vi "Axsun OCT Control Example.vi"() -> ()   [LabVIEW 2018]
uses:
  C:/Projects/Serial Sectioning OCT - TortoiseGIT/SerialSectOCT/Software/Hardware Mfg/Axsun Laser/AxsunOCTControl.dll
  AxsunOCTControl.dll
panel:
  in  "Reg Value (write)":u32 format="%04x"
  out "Reg Value (read)":u16 format="%04x"
  in  "Reg Number":u32
  in  "Write FPGA Register":bool
  in  "Read FPGA Register":bool
  out "Devices":string[](array[string])
  in  "Laser Off":bool
  in  "Laser On":bool
  in  "stop":bool
  out "Error":errorcluster
  out "Version":string
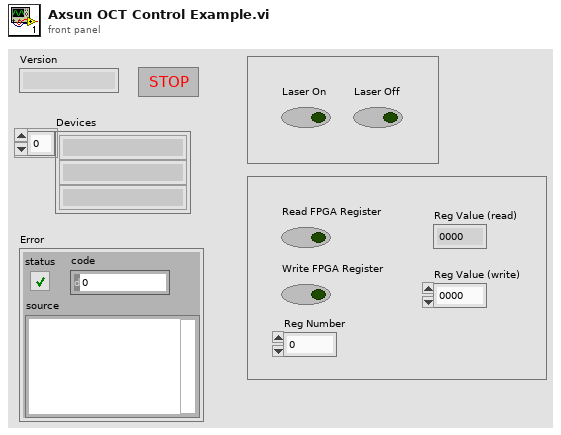
[diagram p1: front panel]
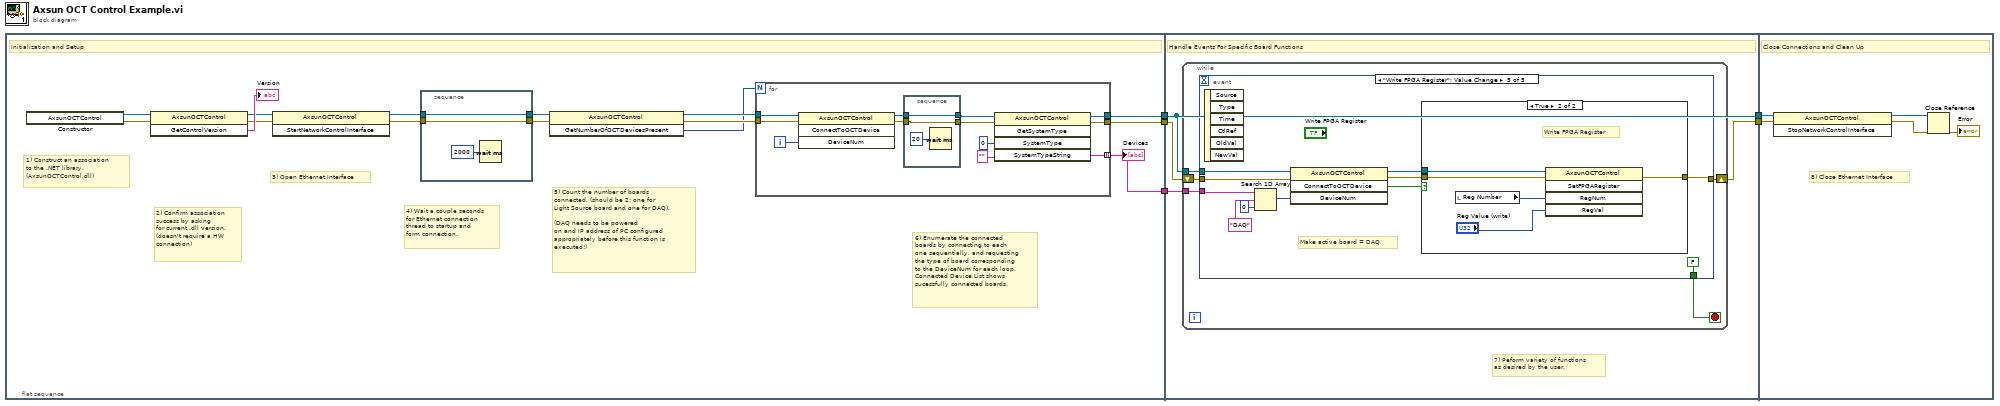
[diagram p0: block diagram]
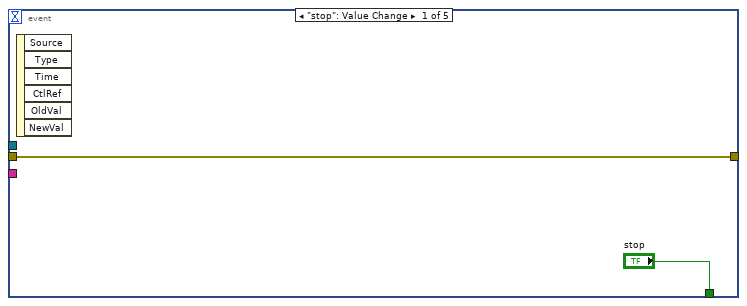
[diagram p2: hidden frame]
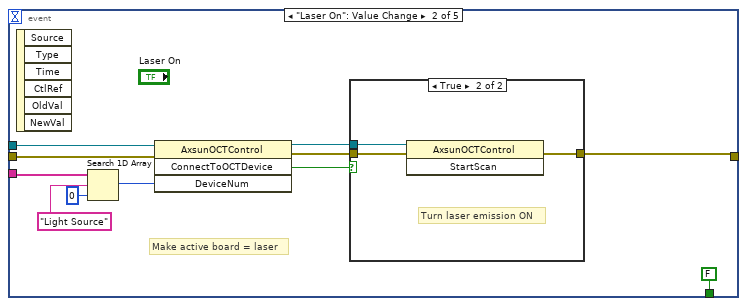
[diagram p3: hidden frame]
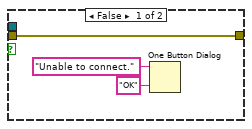
[diagram p4: hidden frame]
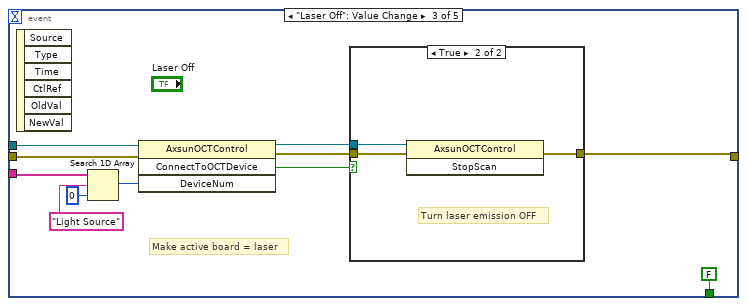
[diagram p5: hidden frame]
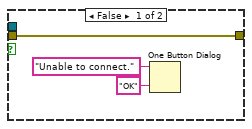
[diagram p6: hidden frame]
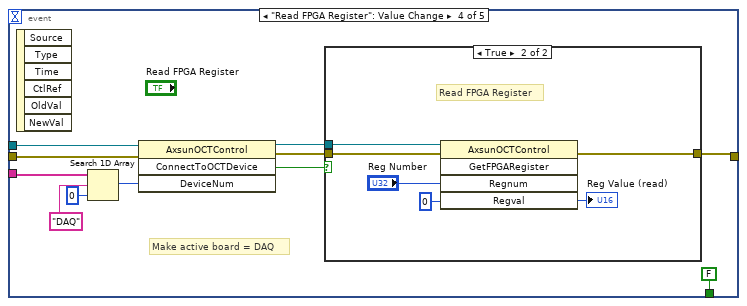
[diagram p7: hidden frame]
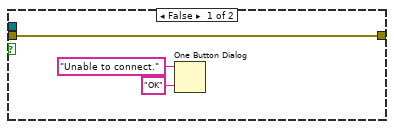
[diagram p8: hidden frame]
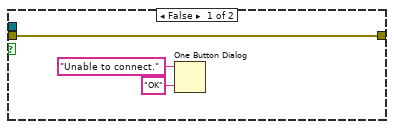
[diagram p9: hidden frame]
diagram:
  n1 = flat-sequence {
    tunnel: [w11] -> w5
    tunnel: [w10] -> w4
    tunnel: [w9] -> w2
    tunnel: w5 -> [w42]
    tunnel: w4 -> [w41]
    tunnel: [w41] -> w3
    tunnel: w2 -> [w40]
    tunnel: [w39] -> w1
    tunnel: w3 -> [w127]
    tunnel: w1 -> [w123]
    frame #0 {
      # "6) Enumerate the connected\nboards by connecting to each\none sequentially, and requesting\nthe type of board corresponding\nto the DeviceNum for each loop.\nConnected Device List shows\nsucessfully connected boards."
      # "5) Count the number of boards\nconnected. (should be 2: one for\nLight Source board and one for DAQ).\n\n(DAQ needs to be powered\non and IP address of PC configured \nappropriately before this function is\nexecuted!)"
      # "4) Wait a couple seconds\nfor Ethernet connection\nthread to startup and\nform connection."
      # "3) Open Ethernet Interface"
      # "2) Confirm association\nsuccess by asking\nfor current .dll version.\n(doesn't require a HW\nconnection)"
      # "1) Construct an association \nto the .NET library.\n(AxsunOCTControl.dll)"
      # "Initialization and Setup"
      n2 = constructor class="AxsunOCTControl"() -> (reference out=w7:refnum<k24>, error out=w6:errorcluster)  [unwired: 3 in, 1 out]
      n3 = invoke class="AxsunOCTControl" method="GetControlVersion"(reference=w7, error in=w6) -> (reference out=w19:refnum<k24>, error out=w18:errorcluster, "GetControlVersion"=→"Version":string)  [unwired: 1 in]
      n4 = invoke class="AxsunOCTControl" method="StartNetworkControlInterface"(reference=w19, error in=w18) -> (reference out=w8:refnum<k24>, error out=w17:errorcluster)  [unwired: 1 in, 1 out]
      n5 = stacked-sequence {
        tunnel: [w38] -> w16
        tunnel: w8 -> [w38]
        tunnel: [w37] -> w15
        tunnel: w17 -> [w37]
        frame #0 {
          n6 = Wait (ms)(milliseconds to wait=u32 2000) -> ()  [unwired: 1 out]
        }
      }
      n7 = invoke class="AxsunOCTControl" method="GetNumberOfOCTDevicesPresent"(reference=w16, error in=w15) -> (reference out=w14:refnum<k24>, error out=w13:errorcluster, "GetNumberOfOCTDevicesPresent"=w12:i32)  [unwired: 1 in]
      n8 = for {
        N: w12 -> [_]
        tunnel: w14 -> [w32]
        tunnel: w13 -> [w31]
        tunnel: [w27] -> w10
        tunnel: [w26] -> w11
        tunnel: [w23] -> w9 mode=indexing
        i -> [w30]
        n9 = invoke class="AxsunOCTControl" method="ConnectToOCTDevice"(reference=w32, error in=w31, "DeviceNum"=w30) -> (reference out=w25:refnum<k24>, error out=w24:errorcluster)  [unwired: 1 in, 2 out]
        n10 = stacked-sequence {
          tunnel: w25 -> [w35]
          tunnel: [w35] -> w22
          tunnel: w24 -> [w34]
          tunnel: [w34] -> w21
          frame #0 {
            n11 = Wait (ms)(milliseconds to wait=u32 20) -> ()  [unwired: 1 out]
          }
        }
        n12 = invoke class="AxsunOCTControl" method="GetSystemType"(reference=w22, error in=w21, "SystemType"=u32 0, "SystemTypeString"="") -> (reference out=w27:refnum<k24>, error out=w26:errorcluster, "SystemTypeString"=w23:string)  [unwired: 1 in, 2 out]
      }
      "Devices" <- w9
    }
    frame #1 {
      # "7) Peform variety of functions\nas desired by the user."
      # "Handle Events For Specific Board Functions"
      n13 = while {
        tunnel: w41 -> [w47]
        tunnel: w40 -> [w44]
        shift-right: [w43] -> w39
        shift-left: w42 -> [w46]
        stop <- w45 stop-if-true
        n14 = event shown="[4] \"Write FPGA Register\": Value Change" {
          selector: _ -> [_ _ _ _ _]
          dyn-events: _ -> [_ _ _ _ _]
          timeout: _ -> [_ _ _ _ _]
          tunnel: w47 -> [_ w57 w74 w91 w111]
          tunnel: w46 -> [w48 w56 w73 w90 w110]
          tunnel: ["stop" FALSE ("stop") FALSE ("stop") FALSE ("stop") FALSE ("stop")] -> w45
          tunnel: w44 -> [_ w59 w76 w93 w113]
          tunnel: [w48 w52 w69 w86 w106] -> w43
          event "stop": Value Change {
            n15 = event-data() -> ()  [unwired: 1 in, 6 out]
          }
          event "Laser On": Value Change {
            # "Make active board = laser"
            n16 = event-data() -> ()  [unwired: 1 in, 6 out]
            n17 = Search 1D Array(1D array=w59, element="Light Source", start index (0)=0) -> (index of element=w55:i32)
            n18 = invoke class="AxsunOCTControl" method="ConnectToOCTDevice"(reference=w57, error in=w56, "DeviceNum"=w55) -> (reference out=w54:refnum<k24>, error out=w53:errorcluster, "ConnectToOCTDevice"=w51:bool)  [unwired: 1 in, 1 out]
            n19 = case shown="True" w51 {
              tunnel: w54 -> [_ w66]
              tunnel: w53 -> [w63 w65]
              tunnel: [w63 w64] -> w52
              frame False {
                n20 = One Button Dialog(message="Unable to connect.", button name ("OK")="OK") -> ()  [unwired: 1 out]
              }
              frame True {
                # "Turn laser emission ON"
                n21 = invoke class="AxsunOCTControl" method="StartScan"(reference=w66, error in=w65) -> (error out=w64:errorcluster)  [unwired: 1 in, 2 out]
              }
            }
          }
          event "Laser Off": Value Change {
            # "Make active board = laser"
            n22 = event-data() -> ()  [unwired: 1 in, 6 out]
            n23 = Search 1D Array(1D array=w76, element="Light Source", start index (0)=0) -> (index of element=w72:i32)
            n24 = invoke class="AxsunOCTControl" method="ConnectToOCTDevice"(reference=w74, error in=w73, "DeviceNum"=w72) -> (reference out=w71:refnum<k24>, error out=w70:errorcluster, "ConnectToOCTDevice"=w68:bool)  [unwired: 1 in, 1 out]
            n25 = case shown="True" w68 {
              tunnel: w71 -> [_ w83]
              tunnel: w70 -> [w80 w82]
              tunnel: [w80 w81] -> w69
              frame False {
                n26 = One Button Dialog(message="Unable to connect.", button name ("OK")="OK") -> ()  [unwired: 1 out]
              }
              frame True {
                # "Turn laser emission OFF"
                n27 = invoke class="AxsunOCTControl" method="StopScan"(reference=w83, error in=w82) -> (error out=w81:errorcluster)  [unwired: 1 in, 2 out]
              }
            }
          }
          event "Read FPGA Register": Value Change {
            # "Make active board = DAQ"
            n28 = event-data() -> ()  [unwired: 1 in, 6 out]
            n29 = Search 1D Array(1D array=w93, element="DAQ", start index (0)=0) -> (index of element=w89:i32)
            n30 = invoke class="AxsunOCTControl" method="ConnectToOCTDevice"(reference=w91, error in=w90, "DeviceNum"=w89) -> (reference out=w88:refnum<k24>, error out=w87:errorcluster, "ConnectToOCTDevice"=w85:bool)  [unwired: 1 in, 1 out]
            n31 = case shown="True" w85 {
              tunnel: w88 -> [_ w103]
              tunnel: w87 -> [w97 w102]
              tunnel: [w97 w101] -> w86
              frame False {
                n32 = One Button Dialog(message="Unable to connect.", button name ("OK")="OK") -> ()  [unwired: 1 out]
              }
              frame True {
                # "Read FPGA Register"
                n33 = invoke class="AxsunOCTControl" method="GetFPGARegister"(reference=w103, error in=w102, "Regnum"="Reg Number", "Regval"=u16 0) -> (error out=w101:errorcluster, "Regval"=→"Reg Value (read)":u16)  [unwired: 1 in, 3 out]
              }
            }
          }
          event "Write FPGA Register": Value Change {
            # "Make active board = DAQ"
            n34 = event-data() -> ()  [unwired: 1 in, 6 out]
            n35 = Search 1D Array(1D array=w113, element="DAQ", start index (0)=0) -> (index of element=w109:i32)
            n36 = invoke class="AxsunOCTControl" method="ConnectToOCTDevice"(reference=w111, error in=w110, "DeviceNum"=w109) -> (reference out=w108:refnum<k24>, error out=w107:errorcluster, "ConnectToOCTDevice"=w105:bool)  [unwired: 1 in, 1 out]
            n37 = case shown="True" w105 {
              tunnel: w108 -> [_ w122]
              tunnel: w107 -> [w117 w121]
              tunnel: [w117 w120] -> w106
              frame False {
                n38 = One Button Dialog(message="Unable to connect.", button name ("OK")="OK") -> ()  [unwired: 1 out]
              }
              frame True {
                # "Write FPGA Register"
                n39 = local read "Reg Number"() -> (w119:u32)
                n40 = invoke class="AxsunOCTControl" method="SetFPGARegister"(reference=w122, error in=w121, "RegNum"=w119, "RegVal"="Reg Value (write)") -> (error out=w120:errorcluster)  [unwired: 1 in, 4 out]
              }
            }
          }
        }
      }
    }
    frame #2 {
      # "8) Close Ethernet Interface"
      # "Close Connections and Clean Up"
      n41 = invoke class="AxsunOCTControl" method="StopNetworkControlInterface"(reference=w127, error in=w123) -> (reference out=w126:refnum<k24>, error out=w125:errorcluster)  [unwired: 1 in, 1 out]
      n42 = Close Reference(reference=w126, error in (no error)=w125) -> (error out=→"Error":errorcluster)
    }
  }
